vi "GetFileListing.vi"(9 "Console In":string) -> (2 "Files":string[](array[string]), 3 "Success?":bool)   [LabVIEW 2016]
uses:
  <vilib>/regexp/Match Regular Expression.xnode
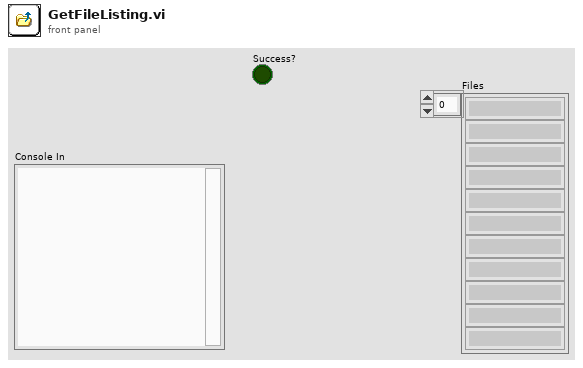
[diagram p1: front panel]
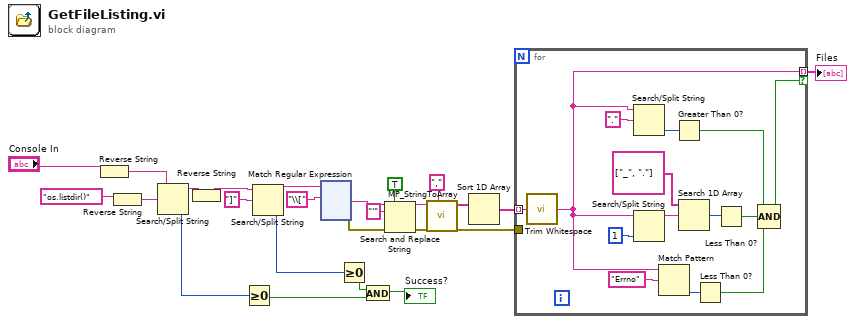
[diagram p0: block diagram]
diagram:
  n1 = Reverse String(1:"Console In") -> (0:w11:string)
  n2 = Reverse String(1:"os.listdir()" ("search string/char (-)")) -> (0:w10:string)
  n3 = Search/Split String(string=w11, search string/char (-)=w10) -> (substring before match=w8:string, offset of match=w4:i32)  [unwired: 1 in, 1 out]
  n4 = Reverse String(1:w8) -> (0:w9:string)
  n5 = Greater Or Equal To 0?(x=w4) -> (x >= 0?=w2:bool)
  n6 = Search/Split String(string=w9, search string/char (-)="]" ("regular expression")) -> (substring before match=w14:string, offset of match=w5:i32)  [unwired: 1 in, 1 out]
  n7 = xnode "Match Regular Expression"("input string"=w14, "regular expression"="\\[") -> ("after match"=w18:string, "error out"=w6:errorcluster)  [unwired: 4 in, 3 out]
  n8 = Greater Or Equal To 0?(x=w5) -> (x >= 0?=w3:bool)
  n9 = And(x=w3, y=w2) -> (x .and. y?=→"Success?":bool)
  n10 = Search and Replace String(replace all?=TRUE ("replace all? (F)"), input string=w18, search string="'", error in=w6) -> (result string=w17:string, error out=w7:errorcluster)  [unwired: 4 in, 2 out]
  n11 = call <userlib>:"MP_StringToArray.vi"("delimiter (LF)"=",", "write buffer"=w17) -> ("Array"=w21:string[])  [unwired: 9 in]
  n12 = Sort 1D Array(array=w21) -> (sorted array=w16:string[])
  n13 = for {
    tunnel: w16 -> [w30] mode=indexing
    tunnel: [w25] -> w15 mode=indexing if=w26
    tunnel: w7 -> [_]
    n14 = call <vilib>:"Trim Whitespace.vi"("string"=w30) -> ("trimmed string"=w25:string)  [unwired: 1 in]
    n15 = Search/Split String(string=w25, search string/char (-)="." ("regular expression")) -> (offset of match=w33:i32)  [unwired: 1 in, 2 out]
    n16 = Search/Split String(string=w25, offset (0)=1) -> (substring before match=w36:string)  [unwired: 1 in, 2 out]
    n17 = Match Pattern(string=w25, regular expression="Errno") -> (offset past match=w31:i32)  [unwired: 1 in, 3 out]
    n18 = Greater Than 0?(x=w33) -> (x > 0?=w27:bool)
    n19 = Search 1D Array(1D array=string[] ["_", "."], element=w36) -> (index of element=w35:i32)  [unwired: 1 in]
    n20 = Less Than 0?(x=w31) -> (x < 0?=w29:bool)
    n21 = Less Than 0?(x=w35) -> (x < 0?=w28:bool)
    n22 = Compound Arithmetic op=AND(w27, w28, w29) -> (w26:bool)
  }
  "Files" <- w15
